vi "_Serial Read Bit.vi"(1 "Port type":u8) -> (0 "BitState":bool)   [LabVIEW 2015]
uses:
  <vilib>/rvi/eio/common/nirviEmuTemplateMethod_errors.vi
  <vilib>/eio/EIOMethodNode/EIOMethodNode.xnode
  <vilib>/eio/EIONode/EIONode.xnode
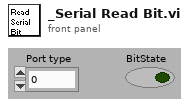
[diagram p1: front panel]
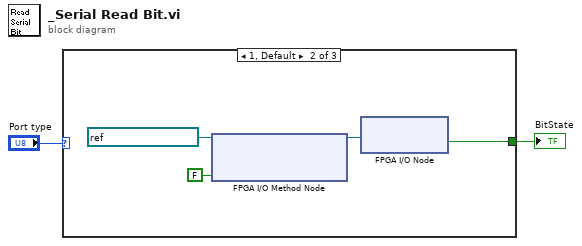
[diagram p0: block diagram]
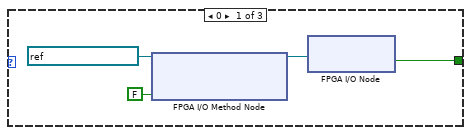
[diagram p2: hidden frame]
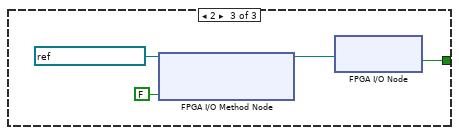
[diagram p3: hidden frame]
diagram:
  n1 = case shown="1, Default" "Port type" {
    tunnel: [w6 w10 w14] -> w2
    frame 0 {
      n2 = xnode "FPGA I/O Method Node"("FPGA I/O In"=refnum<k21> "Digtal IO/DIO46", "Enable"=FALSE) -> ("FPGA I/O Out"=w3:refnum<k21>)
      n3 = xnode "FPGA I/O Node"("FPGA I/O In"=w3) -> ("I/O Item"=w6:bool)  [unwired: 1 out]
    }
    frame 1, Default {
      n4 = xnode "FPGA I/O Method Node"("FPGA I/O In"=refnum<k21> "Digtal IO/DIO44", "Enable"=FALSE) -> ("FPGA I/O Out"=w7:refnum<k21>)
      n5 = xnode "FPGA I/O Node"("FPGA I/O In"=w7) -> ("I/O Item"=w10:bool)  [unwired: 1 out]
    }
    frame 2 {
      n6 = xnode "FPGA I/O Method Node"("FPGA I/O In"=refnum<k21> "Digtal IO/DIO54", "Enable"=FALSE) -> ("FPGA I/O Out"=w13:refnum<k21>)
      n7 = xnode "FPGA I/O Node"("FPGA I/O In"=w13) -> ("I/O Item"=w14:bool)  [unwired: 1 out]
    }
  }
  "BitState" <- w2
